vi "String to DoubleComplex (Scalar).vi"(10 "Value (String)":string) -> (1 "Rest of string":string, 2 "Value (CDB)":cdb format="%#_13g", 3 "offset past number":i32)   [LabVIEW 2013, in "OpenScalar.lvlib"]
uses:
  Get Decimal Separator.vi
  OpenScalar.lvlib
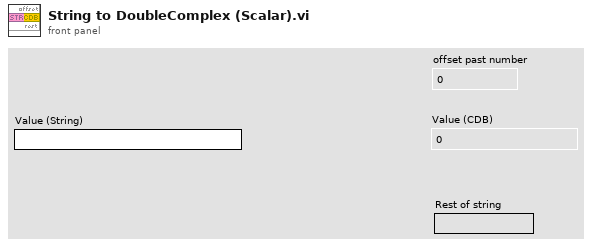
[diagram p1: front panel]
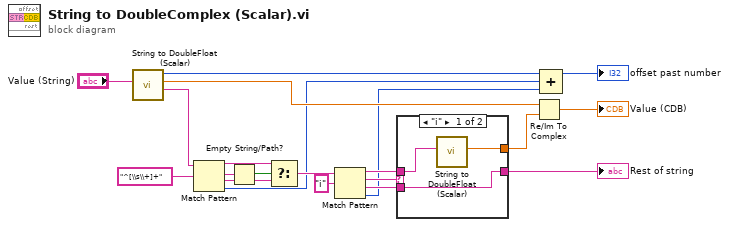
[diagram p0: block diagram]
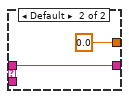
[diagram p2: hidden frame]
diagram:
  n1 = call "String to DoubleFloat (Scalar).vi"("Value (String)"="Value (String)") -> ("Rest of string"=w4:string, "Value (Double)"=w17:dbl, "offset past number"=w12:i32)  [unwired: 8 in]
  n2 = Match Pattern(string=w4, regular expression="^[\\s\\+]+") -> (before substring=w6:string, match substring=w8:string, after substring=w5:string, offset past match=w1:i32)  [unwired: 1 in]
  n3 = Empty String/Path?(string/path=w8) -> (empty?=w7:bool)
  n4 = Select(t=w6, s=w7, f=w5) -> (s? t:f=w3:string)
  n5 = Match Pattern(string=w3, regular expression="i") -> (before substring=w15:string, match substring=w18:string, after substring=w13:string, offset past match=w2:i32)  [unwired: 1 in]
  n6 = case shown="\"i\"" w18 {
    tunnel: [w22 0.0 ("y")] -> w16
    tunnel: w15 -> [w23 w24]
    tunnel: [w21 w24] -> w14
    tunnel: w13 -> [w21 _]
    frame "i" {
      n7 = call "String to DoubleFloat (Scalar).vi"("Value (String)"=w23) -> ("Value (Double)"=w22:dbl)  [unwired: 8 in, 2 out]
    }
    frame Default {
    }
  }
  "Rest of string" <- w14
  n8 = Re/Im To Complex(1:w16, 2:w17) -> (0:→"Value (CDB)":cdb)
  n9 = Compound Arithmetic op=ADD(w12, w1, w2) -> (→"offset past number":i32)
